vi "Writer.vi"   [LabVIEW 2016, in "BTL_logger.lvlib"]
uses:
  BTL_logger.lvlib
  <vilib>/Utility/error.llb/DialogType.ctl
types:
  T1 = enum16{"open", "replace", "create", "open or create", "replace or create", "replace or create with confirmation"}
  T2 = typedef "DialogType.ctl" = u16
  T3 = typedef "BTL_logger.lvlib/Options.ctl" = cluster{"filesize (bytes)":u32, "logs max age (days) ":u16, "write per N messages":u16}
  T4 = typedef "BTL_logger.lvlib/Levels.ctl" = enum16{"ALL", "TRACE", "DEBUG", "INFO", "WARN", "ERROR", "FATAL", "OFF"}
  T5 = typedef "BTL_logger.lvlib/Event.ctl" = cluster{"Time Stamp":timestamp, "Level":T4, "Source":string, "Message":string}
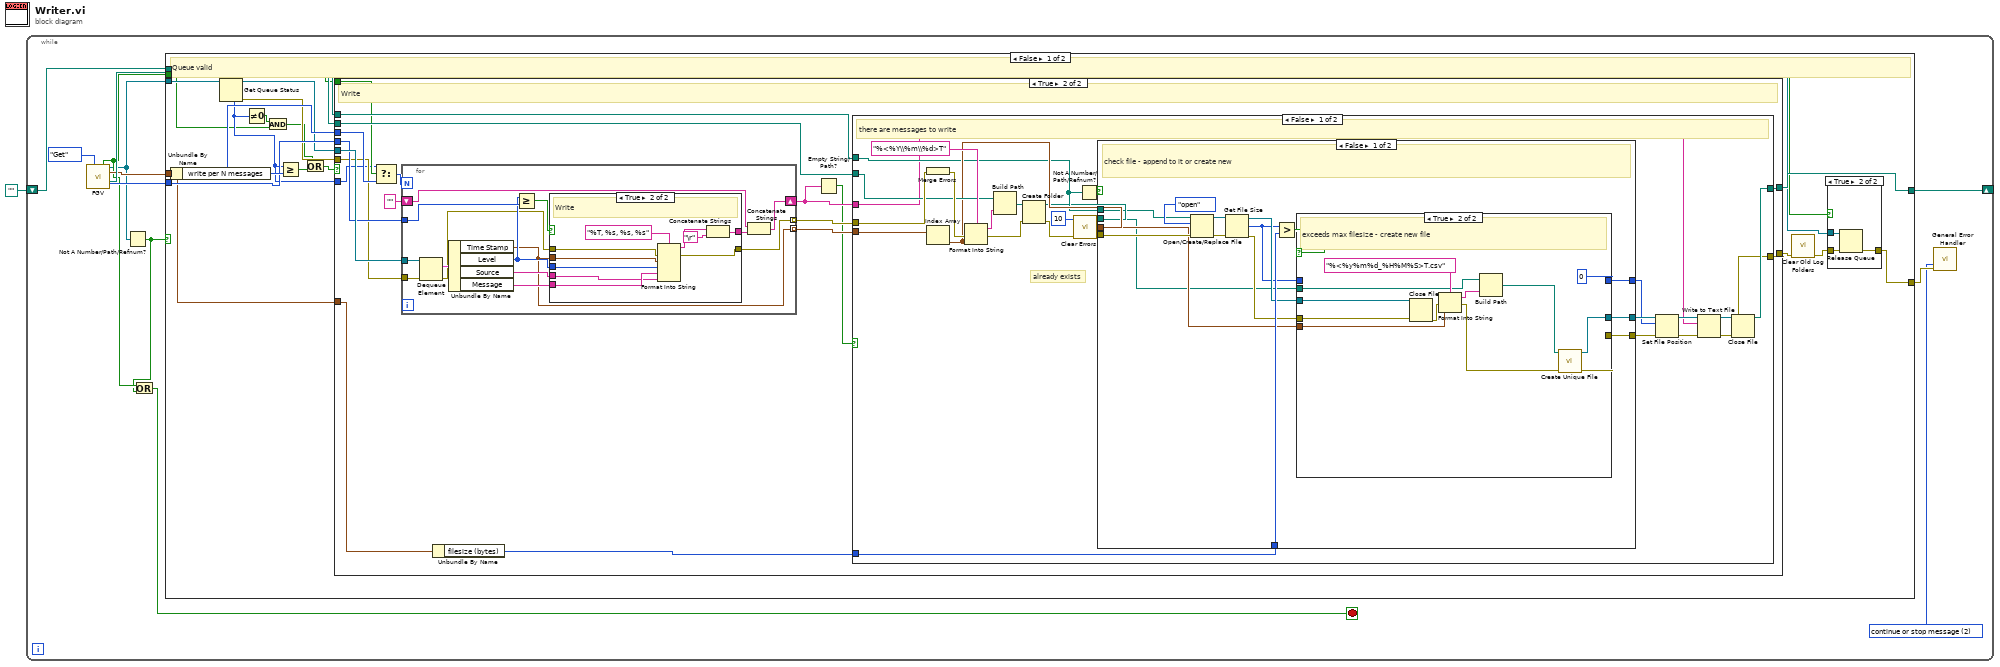
[diagram p0: block diagram]
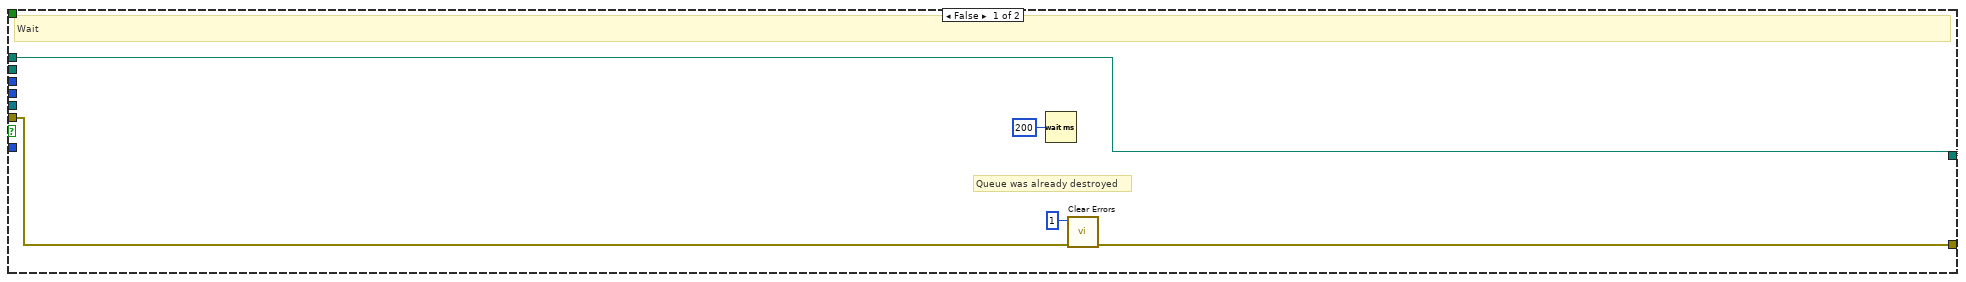
[diagram p3: hidden frame]
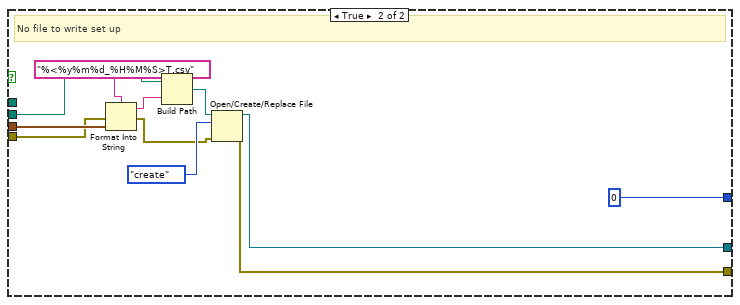
[diagram p5: hidden frame]
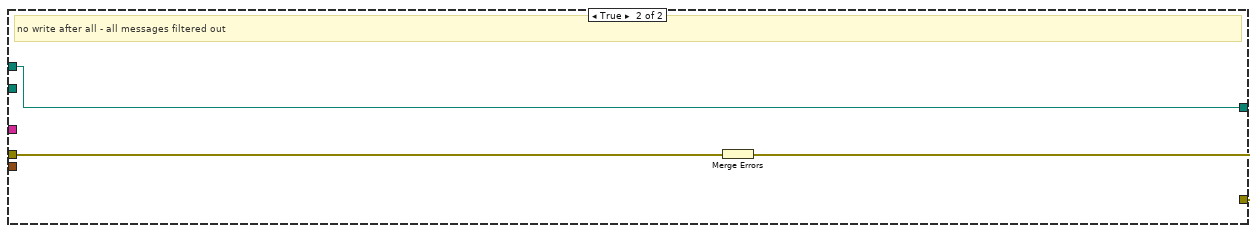
[diagram p6: hidden frame]
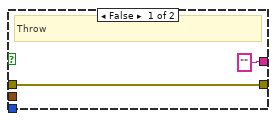
[diagram p7: hidden frame]
diagram:
  n1 = while {
    shift-right: [w10] -> _
    shift-left: path "" -> [w9]
    stop <- w3 stop-if-true
    w4 = T2 2 items=["no dialog", "OK message", "continue or stop message", "OK message + warnings", "continue/stop + warnings"] ("type of dialog (OK msg:1)")
    n2 = call "FGV.vi"("Action"=enum16{"Get", "Set"}."Get") -> ("Destroy Logger out"=w6:bool, "queue out"=w5:refnum<queue>, "Options out"=w8:T3, "Root Logging Path out"=w11:path, "Level out"=w12:T4)  [unwired: 9 in, 1 out]
    n3 = Not A Number/Path/Refnum?(number/path/refnum=w5) -> (NaN/Path/Refnum?=w2:bool)
    n4 = Or(x=w6, y=w2) -> (x .or. y?=w3:bool)
    n5 = case shown="False" w2 {
      tunnel: w12 -> [w29 _]
      tunnel: w11 -> [w27 w155]
      tunnel: [w26 w155] -> w10
      tunnel: w9 -> [w25 _]
      tunnel: w8 -> [w24 _]
      tunnel: [w22 _] -> w7
      tunnel: w6 -> [w14 _]
      tunnel: w5 -> [w15 _]
      frame False {
        # "Queue valid"
        n6 = Unbundle By Name(w24) -> ("write per N messages"=w30:u16)
        n7 = Get Queue Status(queue=w15) -> (queue out=w21:refnum<queue>, error out=w28:errorcluster, # elements in queue=w18:i32)  [unwired: 2 in, 5 out]
        n8 = Not Equal To 0?(x=w18) -> (x != 0?=w17:bool)
        n9 = And(x=w17, y=w14) -> (x .and. y?=w16:bool)
        n10 = Greater Or Equal?(x=w18, y=w30) -> (x >= y?=w31:bool)
        n11 = Or(x=w16, y=w31) -> (x .or. y?=w23:bool)
        n12 = case shown="True" w23 {
          tunnel: w21 -> [_ w58]
          tunnel: w30 -> [_ w57]
          tunnel: w29 -> [_ w56]
          tunnel: w28 -> [w39 w54]
          tunnel: w27 -> [_ w51]
          tunnel: [w40 w47] -> w26
          tunnel: w25 -> [w40 w50]
          tunnel: w24 -> [_ w49]
          tunnel: [w38 w46] -> w20
          tunnel: w14 -> [_ w44]
          tunnel: w18 -> [_ w43]
          frame False {
            # "Queue was already destroyed"
            # "Wait"
            n13 = Wait (ms)(milliseconds to wait=u32 200) -> ()  [unwired: 1 out]
            n14 = call <vilib>:"Clear Errors.vi"("error in (no error)"=w39, "specific error code to clear (0: all)"=1) -> ("error out"=w38:errorcluster)  [unwired: 4 in, 1 out]
          }
          frame True {
            # "Write"
            n15 = Select(t=w43, s=w44, f=w57) -> (s? t:f=w45:i32)
            n16 = for {
              N: w45 -> [_]
              tunnel: w58 -> [w142]
              tunnel: w56 -> [w140]
              shift-right: [w135] -> w42
              shift-left: "" -> [w133]
              tunnel: w54 -> [w132]
              tunnel: [w130] -> w53 mode=indexing
              tunnel: [w129] -> w52 mode=indexing
              n17 = Dequeue Element(queue=w142, error in (no error)=w132) -> (element=w141:T5, error out=w131:errorcluster)  [unwired: 1 in, 2 out]
              n18 = Unbundle By Name(w141) -> ("Time Stamp"=w129:timestamp, "Level"=w138:T4, "Source"=w137:string, "Message"=w136:string)
              n19 = Greater Or Equal?(x=w138, y=w140) -> (x >= y?=w139:bool)
              n20 = case shown="True" w139 {
                tunnel: w129 -> [_ w154]
                tunnel: w138 -> [_ w153]
                tunnel: w137 -> [_ w145]
                tunnel: w136 -> [_ w146]
                tunnel: ["" w149] -> w134
                tunnel: w131 -> [w143 w148]
                tunnel: [w143 w147] -> w130
                frame False {
                  # "Throw"
                }
                frame True {
                  # "Write"
                  n21 = Format Into String(format string="%T, %s, %s, %s", error in=w148, w154, w153, w146, w145) -> (resulting string=w151:string, error out=w147:errorcluster)  [unwired: 1 in]
                  n22 = Concatenate Strings(w151, "\r") -> (w149:string)
                }
              }
              n23 = Concatenate Strings(w133, w134) -> (w135:string)
            }
            n24 = Unbundle By Name(w49) -> ("filesize (bytes)"=w48:u32)
            n25 = Empty String/Path?(string/path=w42) -> (empty?=w41:bool)
            n26 = case shown="False" w41 {
              tunnel: w53 -> [w84 w128]
              tunnel: w52 -> [w83 _]
              tunnel: w51 -> [w80 _]
              tunnel: w50 -> [w74 w126]
              tunnel: w48 -> [w71 _]
              tunnel: [w63 w126] -> w47
              tunnel: [w62 w127] -> w46
              tunnel: w42 -> [w61 _]
              frame False {
                # "already exists"
                # "there are messages to write"
                n27 = Merge Errors(w84) -> (w82:errorcluster)
                n28 = Index Array(array=w83) -> (element=w76:timestamp)  [unwired: 1 in]
                n29 = Format Into String(format string="%<%Y\\%m\\%d>T", error in=w82, w76) -> (resulting string=w79:string, error out=w78:errorcluster)  [unwired: 1 in]
                n30 = Build Path(base path=w80, name or relative path=w79) -> (appended path=w75:path)
                n31 = Create Folder(path (use dialog)=w75, error in=w78) -> (created path=w73:path, error out=w72:errorcluster)  [unwired: 1 in, 1 out]
                n32 = call <vilib>:"Clear Errors.vi"("error in (no error)"=w72, "specific error code to clear (0: all)"=10) -> ("error out"=w60:errorcluster)  [unwired: 4 in, 1 out]
                n33 = Not A Number/Path/Refnum?(number/path/refnum=w74) -> (NaN/Path/Refnum?=w77:bool)
                n34 = case shown="False" w77 {
                  tunnel: w76 -> [w90 w125]
                  tunnel: w73 -> [w89 w124]
                  tunnel: w74 -> [w93 _]
                  tunnel: w60 -> [w97 w122]
                  tunnel: w71 -> [w95 _]
                  tunnel: [w88 w118] -> w68
                  tunnel: [w86 i64 0 ("size (in bytes)")] -> w67
                  tunnel: [w85 w116] -> w66
                  frame False {
                    # "check file - append to it or create new"
                    n35 = Open/Create/Replace File(file path (use dialog)=w93, error in=w97, operation (0:open)=T1."open") -> (refnum out=w99:refnum<file>, error out=w96:errorcluster)  [unwired: 3 in, 1 out]
                    n36 = Get File Size(file=w99, error in=w96) -> (refnum out=w92:refnum<file>, size (in bytes)=w87:i64, 0:w91:errorcluster)
                    n37 = Greater?(x=w87, y=w95) -> (0:w94:bool)
                    n38 = case shown="True" w94 {
                      tunnel: w92 -> [w102 w114]
                      tunnel: w91 -> [w100 w113]
                      tunnel: w90 -> [_ w110]
                      tunnel: w89 -> [_ w103]
                      tunnel: [w102 w105] -> w88
                      tunnel: w87 -> [w101 _]
                      tunnel: [w101 i64 0 ("size (in bytes)")] -> w86
                      tunnel: [w100 w106] -> w85
                      frame False {
                        # "file size is ok"
                      }
                      frame True {
                        # "exceeds max filesize - create new file"
                        n39 = Close File(refnum=w114, error in=w113) -> (error out=w109:errorcluster)  [unwired: 1 out]
                        n40 = Format Into String(format string="%<%y%m%d_%H%M%S>T.csv", error in=w109, w110) -> (resulting string=w112:string, error out=w111:errorcluster)  [unwired: 1 in]
                        n41 = Build Path(base path=w103, name or relative path=w112) -> (appended path=w104:path)
                        n42 = call "Create Unique File.vi"("error in (no error)"=w111, "appended path"=w104) -> ("error out"=w106:errorcluster, "Byte Stream File out"=w105:refnum<file>)  [unwired: 8 in]
                      }
                    }
                  }
                  frame True {
                    # "No file to write set up"
                    n43 = Format Into String(format string="%<%y%m%d_%H%M%S>T.csv", error in=w122, w125) -> (resulting string=w123:string, error out=w119:errorcluster)  [unwired: 1 in]
                    n44 = Build Path(base path=w124, name or relative path=w123) -> (appended path=w121:path)
                    n45 = Open/Create/Replace File(file path (use dialog)=w121, error in=w119, operation (0:open)=T1."create") -> (refnum out=w118:refnum<file>, error out=w116:errorcluster)  [unwired: 3 in, 1 out]
                  }
                }
                n46 = Set File Position(offset (in bytes) (0)=w67, refnum=w68, error in=w66) -> (refnum out=w69:refnum<file>, error out=w65:errorcluster)  [unwired: 1 out]
                n47 = Write to Text File(file (use dialog)=w69, text=w61, error in=w65) -> (refnum out=w70:refnum<file>, error out=w64:errorcluster)  [unwired: 2 out]
                n48 = Close File(refnum=w70, error in=w64) -> (path=w63:path, error out=w62:errorcluster)
              }
              frame True {
                # "no write after all - all messages filtered out"
                n49 = Merge Errors(w128) -> (w127:errorcluster)
              }
            }
          }
        }
        n50 = call "Clear Old Log Folders.vi"("error in (no error)"=w20) -> ("error out"=w19:errorcluster)  [unwired: 10 in]
        n51 = case shown="True" w14 {
          tunnel: [w32 w35] -> w22
          tunnel: w21 -> [_ w34]
          tunnel: w19 -> [w32 w33]
          frame False {
          }
          frame True {
            n52 = Release Queue(queue=w34, error in (no error)=w33) -> (error out=w35:errorcluster)  [unwired: 1 in, 2 out]
          }
        }
      }
      frame True {
        # "Queue invalid"
      }
    }
    n53 = call <vilib>:"General Error Handler.vi"("type of dialog (OK msg:1)"=w4, "error in (no error)"=w7) -> ()  [unwired: 9 in, 5 out]
  }
